vi "SP De-Embed SP.vi"(8 "error in (no error)":errorcluster, 9 "Adapters":T2[](array[typedef]), 10 "SP Array":T3, 11 "Measured Parameters":T4[](array[typedef]) {"Stimulus Port" min=1 step=1; "Response Port" min=1 step=1}) -> (0 "error out":errorcluster, 2 "De-embedded SP Array":T3)   [LabVIEW 2011]
uses:
  TypeDefs/SP Parameter.ctl
  TypeDefs/SP Data.ctl
  TypeDefs/SP Adapter.ctl
  TypeDefs/SP Format.ctl
panel:
  out "S11 VSWR De-embedded":T1(graph)
  out "S21 Log Mag De-embedded":T1(graph)
  out "S21 Log Mag":T1(graph)
  out "S11 VSWR":T1(graph)
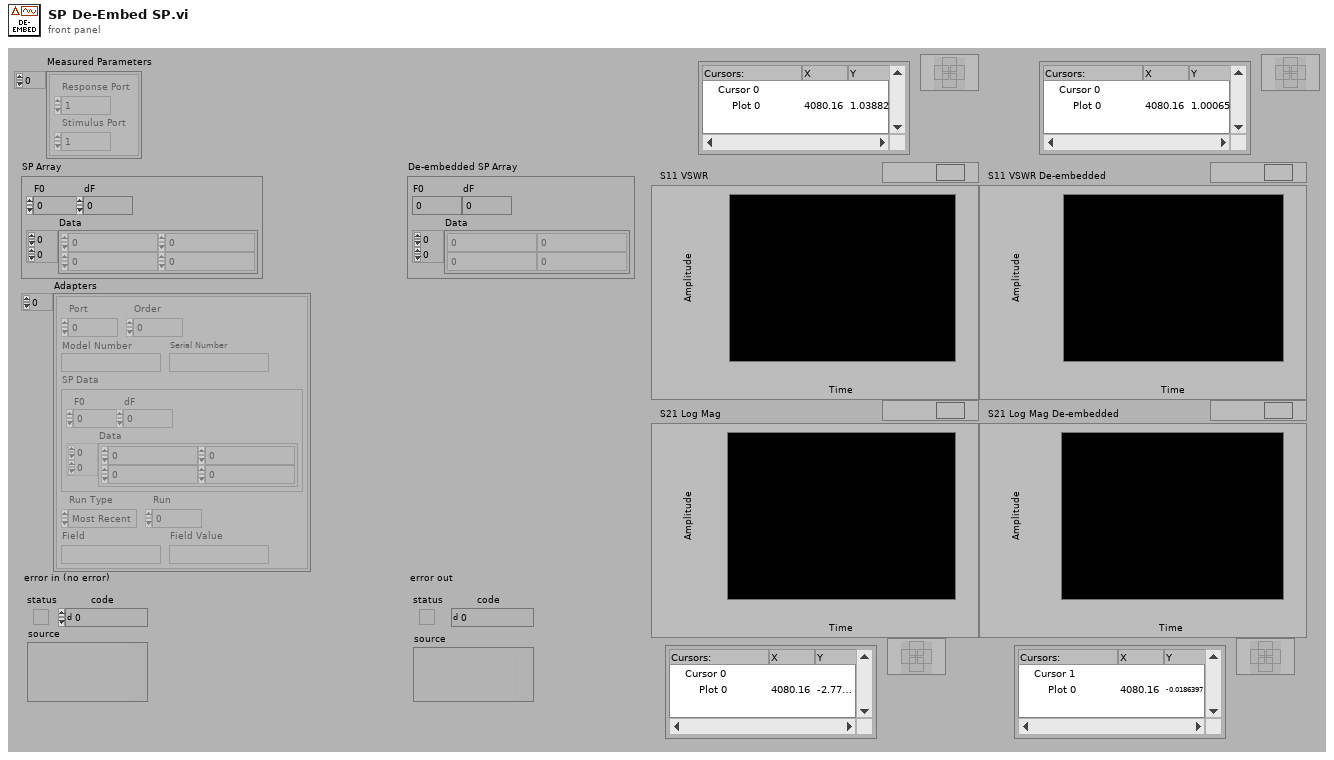
[diagram p1: front panel]
types:
  T1 = cluster{"F0":dbl, "dF":dbl, "Formatted Values":dbl[]}
  T2 = typedef "SP Adapter.ctl" = cluster{"Port":i8, "Order":i8, "Model Number":string, "Serial Number":string, "SP Data":T3, "Run Type":enum16{"Most Recent", "Run #", "Match Field"}, "Run":i32, "Field":string, "Field Value":string}
  T3 = typedef "SP Data.ctl" = cluster{"F0":dbl, "dF":dbl, "Data":cdb[][]}
  T4 = typedef "SP Parameter.ctl" = cluster{"Stimulus Port":i8, "Response Port":i8}
  T5 = typedef "SP Format.ctl" = enum16{"Log Mag", "Lin Mag", "SWR", "Phase", "Expanded Phase", "Delay", "Insertion Loss", "Isolation", "Return Loss"}
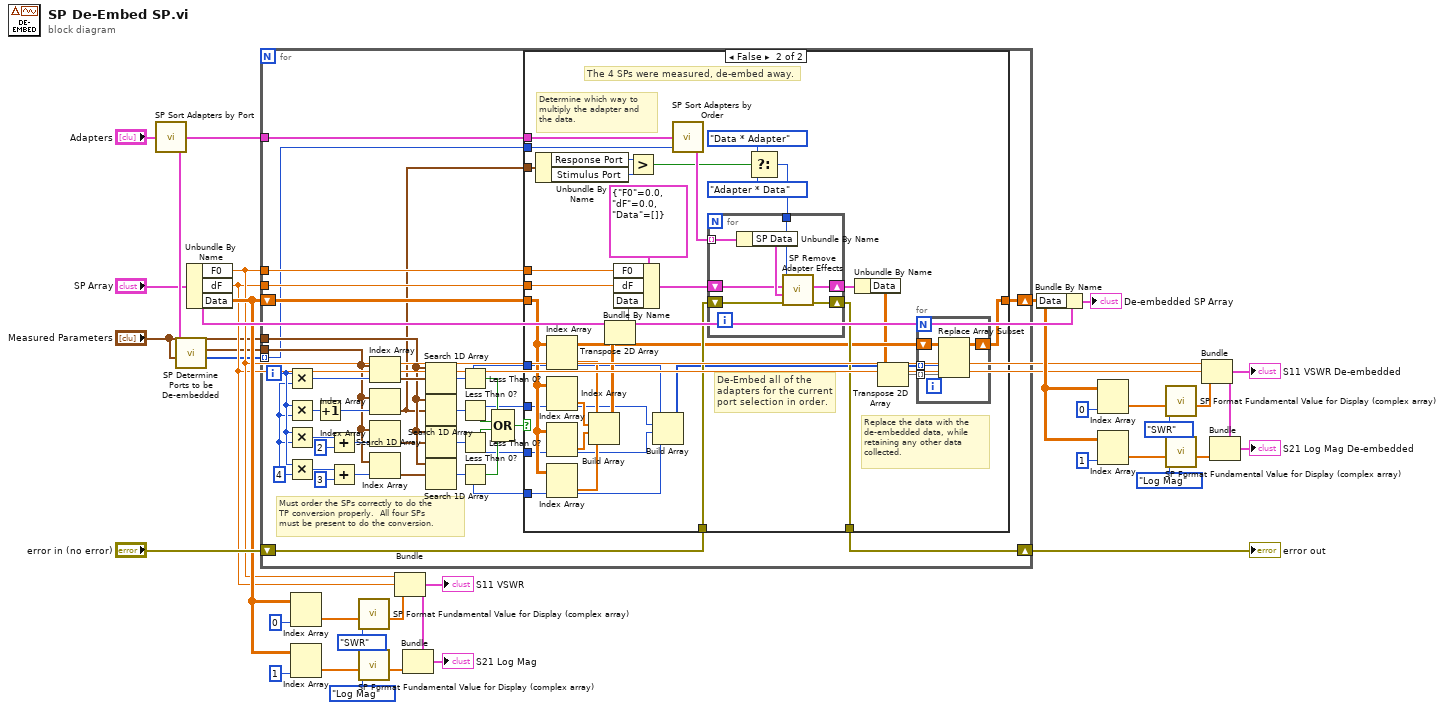
[diagram p0: block diagram]
diagram:
  n1 = call "SP Sort Adapters by Port.vi"("Adapters"="Adapters") -> ("Sorted Adapters"=w32:T2[])
  n2 = call "SP Determine Ports to be De-embedded.vi"("Measured Parameters"="Measured Parameters", "Adapters"=w32) -> ("Ports to De-Embed"=w1:i8[], "Parameters to De-Embed"=w3:T4[])  [unwired: 1 in, 7 out]
  n3 = Unbundle By Name("SP Array") -> ("F0"=w5:dbl, "dF"=w4:dbl, "Data"=w25:cdb[][])
  n4 = for {
    tunnel: w3 -> [w54]
    tunnel: "Measured Parameters" -> [w51]
    shift-right: [w67] -> w6
    shift-left: w25 -> [w66]
    tunnel: w5 -> [w41]
    tunnel: w4 -> [w40]
    tunnel: w32 -> [w39]
    shift-right: [w37] -> w28
    shift-left: "error in (no error)" -> [w38]
    tunnel: w1 -> [w36] mode=indexing
    i -> [w63]
    w59 = 4 ("y")
    # "Must order the SPs correctly to do the\nTP conversion properly.  All four SPs\nmust be present to do the conversion."
    n5 = Multiply(x=w63, y=w59) -> (x*y=w58:i32)
    n6 = Multiply(x=w63, y=w59) -> (x*y=w65:i32)
    n7 = Multiply(x=w63, y=w59) -> (x*y=w64:i32)
    n8 = Multiply(x=w63, y=w59) -> (x*y=w60:i32)
    n9 = Increment(x=w65) -> (x+1=w57:i32)
    n10 = Add(x=w64, y=2) -> (x+y=w56:i32)
    n11 = Add(x=w60, y=3) -> (x+y=w55:i32)
    n12 = Index Array(array=w54, index=w58) -> (element=w53:T4)
    n13 = Index Array(array=w54, index=w57) -> (element=w34:T4)
    n14 = Index Array(array=w54, index=w56) -> (element=w35:T4)
    n15 = Index Array(array=w54, index=w55) -> (element=w52:T4)
    n16 = Search 1D Array(1D array=w51, element=w53) -> (index of element=w45:i32)  [unwired: 1 out]
    n17 = Search 1D Array(1D array=w51, element=w34) -> (index of element=w44:i32)  [unwired: 1 out]
    n18 = Search 1D Array(1D array=w51, element=w35) -> (index of element=w43:i32)  [unwired: 1 out]
    n19 = Search 1D Array(1D array=w51, element=w52) -> (index of element=w42:i32)  [unwired: 1 out]
    n20 = Less Than 0?(x=w45) -> (x < 0?=w50:bool)
    n21 = Less Than 0?(x=w44) -> (x < 0?=w47:bool)
    n22 = Less Than 0?(x=w43) -> (x < 0?=w48:bool)
    n23 = Less Than 0?(x=w42) -> (x < 0?=w49:bool)
    n24 = Compound Arithmetic op=OR(w50, w47, w48, w49) -> (w46:bool)
    n25 = case shown="False" w46 {
      tunnel: w66 -> [w69 w78]
      tunnel: [w69 w70] -> w67
      tunnel: w45 -> [_ w77]
      tunnel: w44 -> [_ w74]
      tunnel: w43 -> [_ w75]
      tunnel: w42 -> [_ w76]
      tunnel: w41 -> [_ w96]
      tunnel: w40 -> [_ w95]
      tunnel: w39 -> [_ w93]
      tunnel: w38 -> [w68 w90]
      tunnel: [w68 w88] -> w37
      tunnel: w36 -> [_ w86]
      tunnel: w34 -> [_ w85]
      frame True {
        # "The 4 SPs were not measured, therefore no de-embedding can be done."
      }
      frame False {
        # "Replace the data with the\nde-embedded data, while\nretaining any other data\ncollected."
        # "De-Embed all of the\nadapters for the current\nport selection in order."
        # "Determine which way to\nmultiply the adapter and\nthe data."
        # "The 4 SPs were measured, de-embed away."
        n26 = Unbundle By Name(w85) -> ("Response Port"=w81:i8, "Stimulus Port"=w80:i8)
        n27 = Index Array(array=w78, index (col)=w77) -> (element=w101:cdb[])  [unwired: 1 in]
        n28 = Index Array(array=w78, index (col)=w74) -> (element=w98:cdb[])  [unwired: 1 in]
        n29 = Index Array(array=w78, index (col)=w75) -> (element=w99:cdb[])  [unwired: 1 in]
        n30 = Index Array(array=w78, index (col)=w76) -> (element=w100:cdb[])  [unwired: 1 in]
        n31 = Build Array(w101, w98, w99, w100) -> (w94:cdb[][])
        n32 = Transpose 2D Array(2D array=w94) -> (transposed array=w89:cdb[][])
        n33 = Bundle By Name(cluster=T3 {"F0"=0.0, "dF"=0.0, "Data"=[]} ("SP Array"), "F0"=w96, "dF"=w95, "Data"=w89) -> (w91:T3)
        n34 = Greater?(x=w81, y=w80) -> (0:w79:bool)
        n35 = Build Array(w77, w74, w75, w76) -> (w73:i32[])
        n36 = call "SP Sort Adapters by Order.vi"("Port"=w86, "Adapters"=w93) -> ("Sorted Adapters"=w92:T2[])  [unwired: 3 out]
        n37 = Select(t=enum16{"Adapter * Data", "Data * Adapter"}."Data * Adapter" ("Multiplication Order"), s=w79, f=enum16{"Adapter * Data", "Data * Adapter"}."Adapter * Data" ("Multiplication Order")) -> (s? t:f=w82:enum16{"Adapter * Data", "Data * Adapter"})
        n38 = for {
          tunnel: w92 -> [w112] mode=indexing
          shift-right: [w109] -> w87
          shift-left: w91 -> [w110]
          shift-right: [w108] -> w88
          shift-left: w90 -> [w107]
          tunnel: w82 -> [w106]
          n39 = Unbundle By Name(w112) -> ("SP Data"=w111:T3)
          n40 = call "SP Remove Adapter Effects.vi"("error in (no error)"=w107, "Adapter S Parameters"=w111, "Data S Parameters"=w110, "Multiplication Order"=w106) -> ("error out"=w108:errorcluster, "New Data  S Parameters"=w109:T3)  [unwired: 6 out]
        }
        n41 = Unbundle By Name(w87) -> ("Data"=w71:cdb[][])
        n42 = Transpose 2D Array(2D array=w71) -> (transposed array=w72:cdb[][])
        n43 = for {
          shift-right: [w104] -> w70
          shift-left: w78 -> [w105]
          tunnel: w73 -> [w103] mode=indexing
          tunnel: w72 -> [w102] mode=indexing
          n44 = Replace Array Subset(array=w105, new element=w102, index (col)=w103) -> (w104:cdb[][])  [unwired: 1 in]
        }
      }
    }
  }
  "error out" <- w28
  n45 = Index Array(array=w25, index (col)=0 ("disabled index (col)")) -> (element=w23:cdb[])  [unwired: 1 in]
  n46 = Index Array(array=w25, index (col)=1 ("disabled index (col)")) -> (element=w21:cdb[])  [unwired: 1 in]
  n47 = call "SP Format Fundamental Value for Display (complex array).vi"("Sxx Measured Format"=SP_Format."SWR" ("Sxx Measure Format"), "Fundamental Values"=w23) -> ("Formatted Values"=w20:dbl[])  [unwired: 1 in, 8 out]
  n48 = call "SP Format Fundamental Value for Display (complex array).vi"("Sxx Measured Format"=SP_Format."Log Mag" ("Sxx Measure Format"), "Fundamental Values"=w21) -> ("Formatted Values"=w18:dbl[])  [unwired: 1 in, 8 out]
  n49 = Bundle("F0"=w5, "dF"=w4, "Formatted Values"=w20) -> (w19:T1)  [unwired: 1 out]
  "S11 VSWR" <- w19
  n50 = Bundle(cluster=w19, "Formatted Values"=w18) -> (→"S21 Log Mag":T1)  [unwired: 2 out]
  n51 = Bundle By Name(cluster="SP Array", "Data"=w6) -> (→"De-embedded SP Array":T3)
  n52 = Index Array(array=w6, index (col)=0 ("disabled index (col)")) -> (element=w10:cdb[])  [unwired: 1 in]
  n53 = Index Array(array=w6, index (col)=1 ("disabled index (col)")) -> (element=w12:cdb[])  [unwired: 1 in]
  n54 = call "SP Format Fundamental Value for Display (complex array).vi"("Sxx Measured Format"=SP_Format."SWR" ("Sxx Measure Format"), "Fundamental Values"=w10) -> ("Formatted Values"=w13:dbl[])  [unwired: 1 in, 8 out]
  n55 = call "SP Format Fundamental Value for Display (complex array).vi"("Sxx Measured Format"=SP_Format."Log Mag" ("Sxx Measure Format"), "Fundamental Values"=w12) -> ("Formatted Values"=w15:dbl[])  [unwired: 1 in, 8 out]
  n56 = Bundle("F0"=w5, "dF"=w4, "Formatted Values"=w13) -> (w14:T1)  [unwired: 1 out]
  "S11 VSWR De-embedded" <- w14
  n57 = Bundle(cluster=w14, "Formatted Values"=w15) -> (→"S21 Log Mag De-embedded":T1)  [unwired: 2 out]
